vi "Adjust Bit Depth (SubVI).vi"(0 "Minimum":u8, 2 "Bit Depth":u8, 5 "Stat. Valid?":bool, 11 "Pixel Data":u8, 12 "Block Size x2":u16, 13 "Pixel Valid?":bool) -> (14 "Output Valid?":bool, 16 "Data Out":u8, 19 "Bid Depth Out":u8)   [LabVIEW 2014]
uses:
  Controls (FPGA)/Sync Block Statistics.ctl
  <vilib>/rvi/Emulation/niFpgaSctlEmulationGetInTimedLoop.vi
  <vilib>/Utility/error.llb/Clear Errors.vi
  <vilib>/rvi/DataTransferAndStorage/Container/Common/niFpgaContainerGetUniqueNameForEmu.vi
  <vilib>/rvi/DataTransferAndStorage/Container/Common/niFpgaContainerSetEmuInfo.vi
  <vilib>/rvi/eio/common/nirviEmuReportErrorAndStop.vi
  <vilib>/rvi/Emulation/niFpgaEmulationIsFPGAContextNoSignature.vi
  <vilib>/rvi/errors/niFpgaSetErrorForExecOnDevCompSimple.vi
  <vilib>/rvi/FIFO/Fifo_Resource/nirvififoEmulationSetSize.vi
  <vilib>/rvi/FIFO/Fifo_Resource/nirviFifoEmulationQueueMgr.vi
  <instcachedir>/0/nirviFifoEmulationQueueMgr_E5CAEC123FF24DC58D834DCA3CDAA9B5.lvgen/nirviFifoEmulationQueueMgr_E5CAEC123FF24DC58D834DCA3CDAA9B5_001.vi
  <vilib>/rvi/FIFO/Fifo_Resource/nirvififoEmulationDetermineInputValidOut.vi
  <vilib>/rvi/FIFO/Fifo_Resource/nirvififoEmulationCreateLock.vi
  <vilib>/rvi/Emulation/niFpgaProcessEmulError.vi
  <vilib>/rvi/FIFO/Fifo_Resource/nirvififoEmulationObtainLock.vi
  <vilib>/rvi/FIFO/Fifo_Resource/nirvififoEmulationReleaseLock.vi
  <vilib>/rvi/occurrence/nirviWaitOnOccurrenceBase.vi
  <vilib>/rvi/errors/nirviReportUnexpectedCaseInternalError.vi
  <vilib>/rvi/errors/nirviReportUnexpectedCaseInternalError (U32).vi
  <instcachedir>/0/nirviFifoEmulationQueueMgr_E5CAEC123FF24DC58D834DCA3CDAA9B5.lvgen/nirviFifoEmulationQueueMgr_E5CAEC123FF24DC58D834DCA3CDAA9B5_003.vi
  <vilib>/rvi/LocalResourceManager/LocalResourceManager.xnode
  <vilib>/rvi/DataTransferAndStorage/Container/XNode/niFpgaContainer.xnode
  <vilib>/rvi/FIFO/Fifo_Resource/nirvififoEmulationWrite.vi
  <vilib>/rvi/FIFO/Fifo_Resource/nirvififoEmulationRead.vi
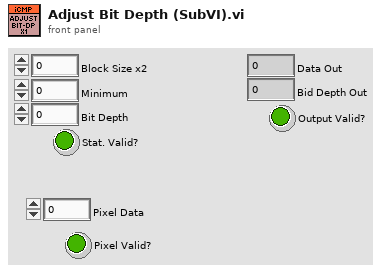
[diagram p1: front panel]
types:
  T1 = typedef "Sync Block Statistics.ctl" = enum16{"Wait for Start", "Wait for End"}
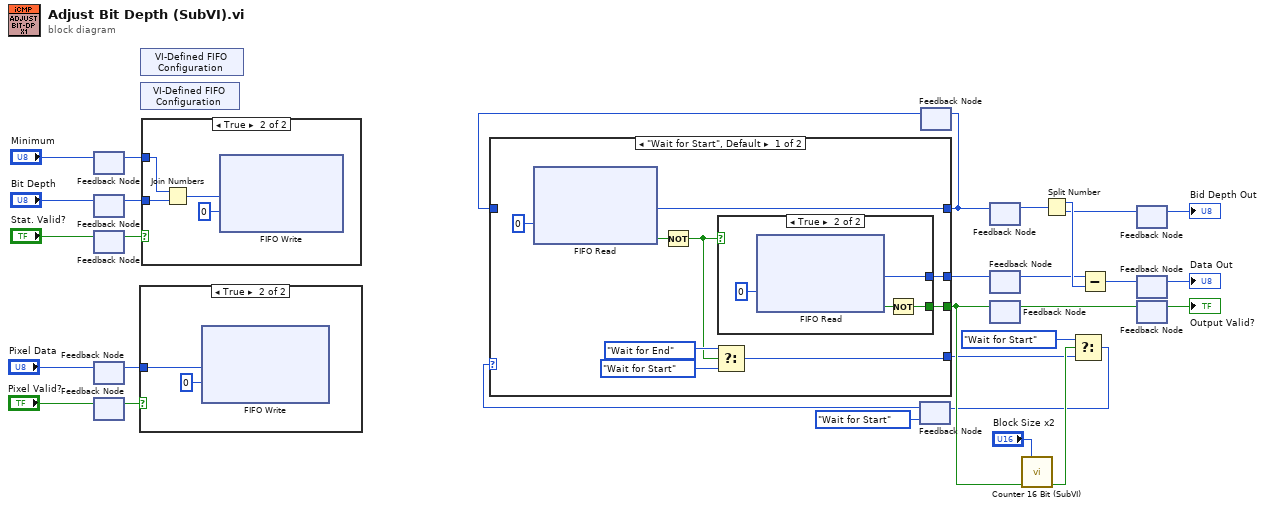
[diagram p0: block diagram]
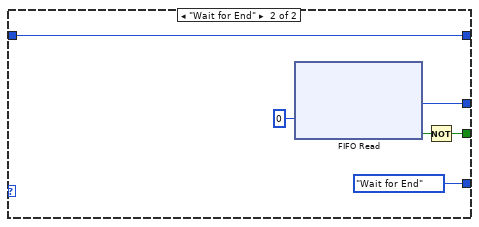
[diagram p3: hidden frame]
diagram:
  n1 = feedback-in #1("Minimum") -> ()
  n2 = feedback #1() -> (w5:u8)  [unwired: 1 in]
  n3 = feedback-in #2("Bit Depth") -> ()
  n4 = feedback #2() -> (w4:u8)  [unwired: 1 in]
  n5 = feedback-in #3("Stat. Valid?") -> ()
  n6 = feedback #3() -> (w3:bool)  [unwired: 1 in]
  n7 = feedback-in #4("Pixel Data") -> ()
  n8 = feedback #4() -> (w2:u8)  [unwired: 1 in]
  n9 = feedback-in #5("Pixel Valid?") -> ()
  n10 = feedback #5() -> (w1:bool)  [unwired: 1 in]
  n11 = case shown="True" w1 {
    tunnel: w2 -> [_ w31]
    frame False {
    }
    frame True {
      n12 = xnode "FIFO Write"("Element"=w31, "Timeout"=0) -> ()  [unwired: 1 in, 2 out]
    }
  }
  n13 = xnode "VI-Defined FIFO Configuration"() -> ()  [unwired: 1 out]
  n14 = xnode "VI-Defined FIFO Configuration"() -> ()  [unwired: 1 out]
  n15 = case shown="True" w3 {
    tunnel: w5 -> [_ w34]
    tunnel: w4 -> [_ w33]
    frame False {
    }
    frame True {
      n16 = Join Numbers(hi=w34, lo=w33) -> ((hi.lo)=w35:u16)
      n17 = xnode "FIFO Write"("Element"=w35, "Timeout"=0) -> ()  [unwired: 1 in, 2 out]
    }
  }
  n18 = feedback #6(Sync_Block_Statistics."Wait for Start" ("Sync Block Statistics")) -> (w25:T1)
  n19 = feedback #7() -> (w23:u16)  [unwired: 1 in]
  n20 = case shown="\"Wait for Start\", Default" w25 {
    tunnel: [w43 Sync_Block_Statistics."Wait for End" ("Sync Block Statistics")] -> w18
    tunnel: [w40 w50] -> w22
    tunnel: [w38 w54] -> w16
    tunnel: w23 -> [_ w54]
    tunnel: [w37 w51] -> w15
    frame "Wait for Start", Default {
      n21 = xnode "FIFO Read"("Timeout"=0) -> ("Element"=w38:u16, "Timed Out?"=w41:bool)  [unwired: 1 in, 1 out]
      n22 = Not(x=w41) -> (.not. x?=w39:bool)
      n23 = Select(t=Sync_Block_Statistics."Wait for End" ("Sync Block Statistics"), s=w39, f=Sync_Block_Statistics."Wait for Start" ("Sync Block Statistics")) -> (s? t:f=w43:T1)
      n24 = case shown="True" w39 {
        tunnel: [_ w47] -> w40
        tunnel: [_ w46] -> w37
        frame False {
        }
        frame True {
          n25 = xnode "FIFO Read"("Timeout"=0) -> ("Element"=w46:u8, "Timed Out?"=w48:bool)  [unwired: 1 in, 1 out]
          n26 = Not(x=w48) -> (.not. x?=w47:bool)
        }
      }
    }
    frame "Wait for End" {
      n27 = xnode "FIFO Read"("Timeout"=0) -> ("Element"=w51:u8, "Timed Out?"=w53:bool)  [unwired: 1 in, 1 out]
      n28 = Not(x=w53) -> (.not. x?=w50:bool)
    }
  }
  n29 = feedback-in #7(w16) -> ()
  n30 = feedback-in #8(w16) -> ()
  n31 = feedback #8() -> (w11:u16)  [unwired: 1 in]
  n32 = feedback-in #9(w15) -> ()
  n33 = feedback #9() -> (w10:u8)  [unwired: 1 in]
  n34 = feedback-in #10(w22) -> ()
  n35 = feedback #10() -> (w9:bool)  [unwired: 1 in]
  n36 = call "Counter 16 Bit (SubVI).vi"("Max. Count"="Block Size x2", "Enable"=w22) -> ("Count End?"=w19:bool)  [unwired: 11 in, 2 out]
  n37 = Split Number(x=w11) -> (hi(x)=w14:u8, lo(x)=w13:u8)
  n38 = Select(t=Sync_Block_Statistics."Wait for Start" ("Sync Block Statistics"), s=w19, f=w18) -> (s? t:f=w17:T1)
  n39 = feedback-in #6(w17) -> ()
  n40 = Subtract(x=w10, y=w14) -> (x-y=w12:u8)
  n41 = feedback-in #11(w13) -> ()
  n42 = feedback #11() -> (→"Bid Depth Out":u8)  [unwired: 1 in]
  n43 = feedback-in #12(w12) -> ()
  n44 = feedback #12() -> (→"Data Out":u8)  [unwired: 1 in]
  n45 = feedback-in #13(w9) -> ()
  n46 = feedback #13() -> (→"Output Valid?":bool)  [unwired: 1 in]
